vi "string2value.vi"(2 "variables":dbl[](array[numeric])=[0.6492890995260664, 0.6502542857506003], 3 "String":string="v1*2") -> (1 "value":dbl)   [LabVIEW 2011]
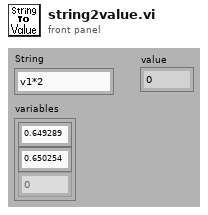
[diagram p1: front panel]
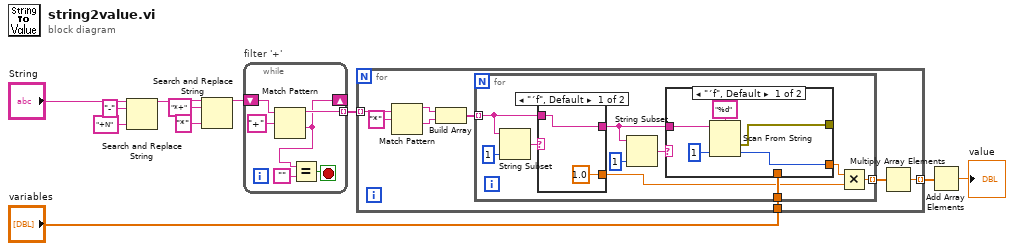
[diagram p0: block diagram]
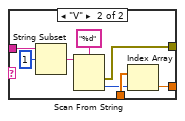
[diagram p2: hidden frame]
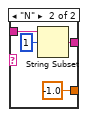
[diagram p3: hidden frame]
diagram:
  n1 = Search and Replace String(input string="String", search string="-", replace string="+N" ("replace string (\"\")")) -> (result string=w7:string)  [unwired: 5 in, 3 out]
  n2 = Search and Replace String(input string=w7, search string="*+", replace string="*" ("replace string (\"\")")) -> (result string=w10:string)  [unwired: 5 in, 3 out]
  n3 = while "filter '+'" {
    tunnel: [w15] -> w11 mode=indexing
    shift-right: [w12] -> _
    shift-left: w10 -> [w16]
    stop <- w14 stop-if-true
    n4 = Match Pattern(string=w16, regular expression="+") -> (before substring=w15:string, after substring=w12:string)  [unwired: 1 in, 2 out]
    n5 = Equal?(x=w12, y="") -> (x = y?=w14:bool)
  }
  n6 = for {
    tunnel: w11 -> [w25] mode=indexing
    tunnel: "variables" -> [w20]
    tunnel: [w18] -> w2 mode=indexing
    n7 = Match Pattern(string=w25, regular expression="*") -> (before substring=w22:string, after substring=w23:string)  [unwired: 1 in, 2 out]
    n8 = Build Array(w22, w23) -> (w21:string[])
    n9 = for {
      tunnel: w21 -> [w33] mode=indexing
      tunnel: [w26] -> w19 mode=indexing
      tunnel: w20 -> [w29]
      n10 = String Subset(string=w33, length (rest)=1 ("length (rest)")) -> (substring=w34:string)  [unwired: 1 in]
      n11 = case shown="\"´f\", Default" w34 {
        tunnel: w33 -> [w49 w54]
        tunnel: [w49 w52] -> w30
        tunnel: [1.0 ("t") -1.0 ("t")] -> w28
        frame "´f", Default {
        }
        frame "N" {
          n12 = String Subset(string=w54, offset (0)=1) -> (substring=w52:string)  [unwired: 1 in]
        }
      }
      n13 = String Subset(string=w30, length (rest)=1 ("length (rest)")) -> (substring=w31:string)  [unwired: 1 in]
      n14 = case shown="\"´f\", Default" w31 {
        tunnel: w30 -> [w40 w48]
        tunnel: [w37 w42] -> _
        tunnel: w29 -> [_ w44]
        tunnel: [w38 w41] -> w27
        frame "´f", Default {
          n15 = Scan From String(format string="%d", input string=w40, default 1=1 ("default value 1")) -> (error out=w37:errorcluster, output 1=w38:i32)  [unwired: 2 in, 2 out]
        }
        frame "V" {
          n16 = String Subset(string=w48, offset (0)=1) -> (substring=w46:string)  [unwired: 1 in]
          n17 = Scan From String(format string="%d", input string=w46) -> (error out=w42:errorcluster, output 1=w43:i32)  [unwired: 3 in, 2 out]
          n18 = Index Array(array=w44, index=w43) -> (element=w41:dbl)
        }
      }
      n19 = Multiply(x=w27, y=w28) -> (x*y=w26:dbl)
    }
    n20 = Multiply Array Elements(1:w19) -> (0:w18:dbl)
  }
  n21 = Add Array Elements(numeric array=w2) -> (sum=→"value":dbl)
